vi "Read Description.vi"(8 "error in (no error)":errorcluster, 11 "Base Interface in":refnum<class "Base Interface.lvclass">) -> (0 "error out":errorcluster, 2 "description":string, 3 "Base Interface out":refnum<class "Base Interface.lvclass">)   [LabVIEW 2020, in "PV Access.lvlib" / "PV Data.lvlib" / "Base Interface.lvclass"]
uses:
  Base Interface.lvclass
  5501c30b-6b64-430b-aa5d-769511abe6e8.vi
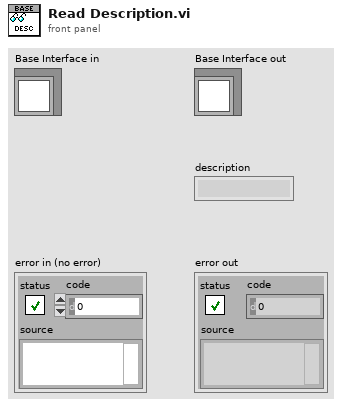
[diagram p1: front panel]
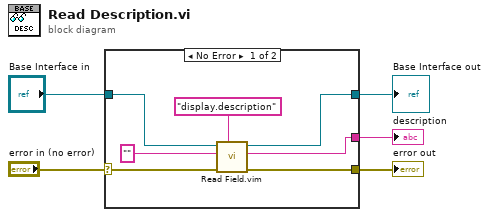
[diagram p0: block diagram]
diagram:
  n1 = case shown="No Error" "error in (no error)" {
    selector: "error in (no error)" -> [w9 w14]
    tunnel: [w8 w14] -> w4
    tunnel: [w11 w13] -> w2
    tunnel: "Base Interface in" -> [w12 w13]
    tunnel: [w6 _] -> w1
    frame No Error {
      n2 = call "Read Field.vim"("field"="display.description", "error in"=w9, "default value"="", "Base Interface in"=w12) -> ("error out"=w8:errorcluster, "value"=w6:string, "Base Interface out"=w11:refnum<class "Base Interface.lvclass">)  [unwired: 5 in]
    }
    frame Error {
    }
  }
  "error out" <- w4
  "Base Interface out" <- w2
  "description" <- w1
